vi "CheckCRC.vi"(8 "error in (no error)":errorcluster, 10 "CRC":u32, 11 "File Size":i32) -> (0 "error out":errorcluster, 2 "Tag Name":string, 3 "Found?":bool)   [LabVIEW 2024]
uses:
  <vilib>/Utility/config.llb/Read Key (I32).vi
  <vilib>/Utility/config.llb/Read Key (U32).vi
  <vilib>/Utility/config.llb/NI_LVConfig.lvlib
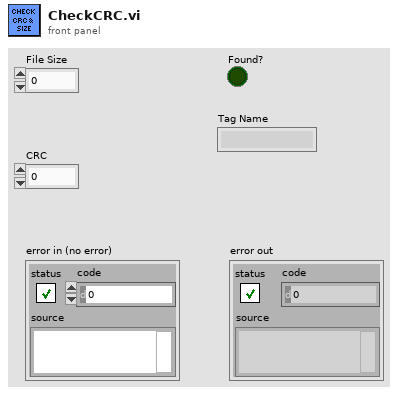
[diagram p1: front panel]
types:
  T1 = typedef "NI_LVConfig.lvlib/Config Data RefNum.ctl" = refnum<k1>
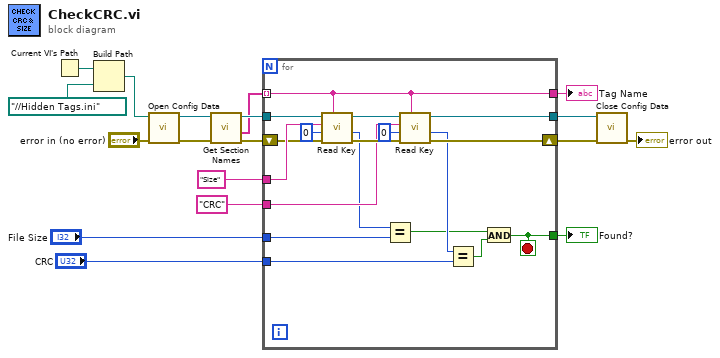
[diagram p0: block diagram]
diagram:
  n1 = Current VI's Path() -> (path=w15:path)
  n2 = Build Path(base path=w15, name or relative path=path "../../Hidden Tags.ini") -> (appended path=w17:path)
  n3 = call <vilib>:"Open Config Data.vi"("error in (no error)"="error in (no error)", "configuration file path"=w17) -> ("error out"=w13:errorcluster, "refnum"=w14:T1)  [unwired: 7 in, 1 out]
  n4 = call <vilib>:"Get Section Names.vi"("error in (no error)"=w13, "refnum"=w14) -> ("error out"=w6:errorcluster, "section names"=w11:string[], "refnum out"=w12:T1)  [unwired: 7 in]
  n5 = for {
    tunnel: w12 -> [w36]
    tunnel: w11 -> [w19] mode=indexing
    tunnel: "Size" -> [w33]
    tunnel: "CRC" -> [w32]
    tunnel: "File Size" -> [w28]
    shift-right: [w27] -> w7
    shift-left: w6 -> [w26]
    tunnel: "CRC" -> [w24]
    tunnel: [w21] -> w4
    tunnel: [w20] -> w3
    tunnel: [w19] -> w1
    stop <- w21 stop-if-true
    n6 = call-poly <vilib>:"Read Key.vi"("section"=w19, "error in (no error)"=w26, "default value"=0, "key"=w33, "refnum"=w36) -> ("error out"=w34:errorcluster, "value"=w29:i32, "refnum out"=w35:T1)  [unwired: 3 in, 1 out]
    n7 = Equal?(x=w29, y=w28) -> (x = y?=w22:bool)
    n8 = call-poly <vilib>:"Read Key.vi"("section"=w19, "error in (no error)"=w34, "default value"=u32 0, "key"=w32, "refnum"=w35) -> ("error out"=w27:errorcluster, "value"=w25:u32, "refnum out"=w20:T1)  [unwired: 3 in, 1 out]
    n9 = Equal?(x=w25, y=w24) -> (x = y?=w23:bool)
    n10 = And(x=w22, y=w23) -> (x .and. y?=w21:bool)
  }
  "Found?" <- w4
  "Tag Name" <- w1
  n11 = call <vilib>:"Close Config Data.vi"("error in (no error)"=w7, "refnum"=w3) -> ("error out"=→"error out":errorcluster)  [unwired: 8 in, 1 out]
